vi "WSVCAP SHL Host TL I2C Write - Single Device.vi"(0 "Sub Address [U8]":u8=20 format="%.0x", 3 "FPGA":T1, 5 "Data Out [U8]":u8=20 format="%.0x", 11 "error in":errorcluster, 12 "DUT":T2, 14 "Log (T)":bool=TRUE) -> (15 "error out":errorcluster)   [LabVIEW 2017]
uses:
  Type Defs/WSVCAP SHL DUT Number Enum.ctl
  Type Defs/WSVCAP SHL FPGA Enum.ctl
panel:
  out "Socket Mask Set [U64]":u64 format="%012x"
  out "C Data Out [U8]":u8[](array[numeric]) format="%.0x"
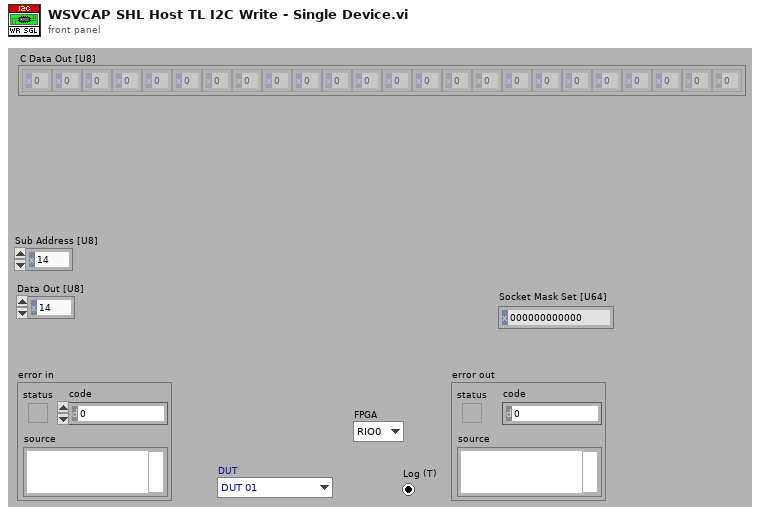
[diagram p1: front panel]
types:
  T1 = typedef "WSVCAP SHL FPGA Enum.ctl" = enum16{"RIO0", "RIO1"}
  T2 = typedef "WSVCAP SHL DUT Number Enum.ctl" = enum16{"DUT 01", "DUT 02", "DUT 03", "DUT 04", "DUT 05", "DUT 06", "DUT 07", "DUT 08", "DUT 09", "DUT 10", "DUT 11", "DUT 12", "DUT 13", "DUT 14", "DUT 15", "DUT 16", "DUT 17", "DUT 18", "DUT 19", "DUT 20", "DUT 21", "DUT 22", "DUT 23", "DUT 24", "DUT 25", "DUT 26", "DUT 27", "DUT 28", "DUT 29", "DUT 30", "DUT 31", "DUT 32", "DUT 33", "DUT 34", "DUT 35", "DUT 36", "DUT 37", "DUT 38", "DUT 39", "DUT 40", "DUT 41", "DUT 42", "DUT 43", "DUT 44", "DUT 45", "DUT 46", "DUT 47", "DUT 48", "DUT 49", "DUT 50", "DUT 51", "DUT 52", "DUT 53", "DUT 54", "DUT 55", "DUT 56", "DUT 57", "DUT 58", "DUT 59", "DUT 60", "DUT 61", "DUT 62", "DUT 63", "DUT 64"}
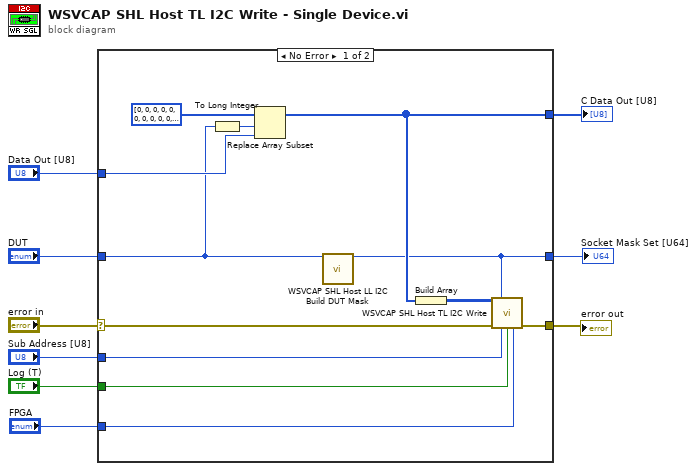
[diagram p0: block diagram]
diagram:
  n1 = case shown="No Error" "error in" {
    selector: "error in" -> [w15 w22]
    tunnel: [w21 w22] -> w9
    tunnel: "Sub Address [U8]" -> [w13 _]
    tunnel: "Data Out [U8]" -> [w20 _]
    tunnel: [w18 _] -> w5
    tunnel: "DUT" -> [w17 _]
    tunnel: [w11 _] -> w3
    tunnel: "Log (T)" -> [w14 _]
    tunnel: "FPGA" -> [w12 _]
    frame No Error {
      n2 = To Long Integer(number=w17) -> (32bit integer=w19:i32)
      n3 = Replace Array Subset(array=u8[] [0, 0, 0, 0, 0, 0, 0, 0, 0, 0, 0, 0, 0, 0, 0, 0, 0, 0, 0, 0, 0, 0, 0, 0, 0, 0, 0, 0, 0, 0, 0, 0, 0, 0, 0, 0, 0, 0, 0, 0, 0, 0, 0, 0, 0, 0, 0, 0, 0, 0, 0, 0, 0, 0, 0, 0, 0, 0, 0, 0, 0, 0, 0, 0] ("SPI Data Out"), new element=w20, index=w19) -> (w18:u8[])
      n4 = call "WSVCAP SHL Host LL I2C Build DUT Mask.vi"("DUT"=w17) -> ("Socket Mask [U64]"=w11:u64)  [unwired: 13 in, 1 out]
      n5 = Build Array(w18) -> (w16:u8[][])
      n6 = call "WSVCAP SHL Host TL I2C Write.vi"("C Data Out"=w16, "Socket Mask [U64]"=w11, "error in"=w15, "Sub Address"=w13, "Log (T)"=w14, "FPGA"=w12) -> ("error out"=w21:errorcluster)  [unwired: 9 in]
    }
    frame Error {
    }
  }
  "error out" <- w9
  "C Data Out [U8]" <- w5
  "Socket Mask Set [U64]" <- w3
